vi "Unwrap Heading.vi"(11 "input":T1[](array[typedef])) -> (3 "output":T1[](array[typedef]))   [LabVIEW 2016]
uses:
  VIs/Segment.ctl
  <vilib>/ptbypt/NI_PtbyPt.lvlib
  Pathfinder.lvlib
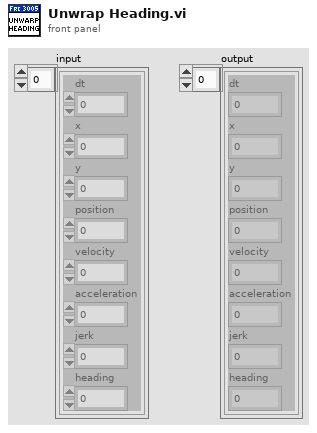
[diagram p1: front panel]
types:
  T1 = typedef "Pathfinder.lvlib/Segment.ctl" = cluster{"dt":dbl, "x":dbl, "y":dbl, "position":dbl, "velocity":dbl, "acceleration":dbl, "jerk":dbl, "heading":dbl}
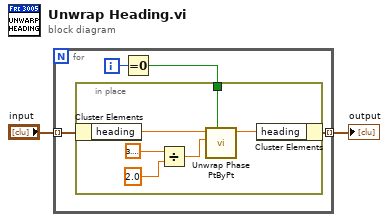
[diagram p0: block diagram]
diagram:
  n1 = for {
    tunnel: "input" -> [w6] mode=indexing
    tunnel: [w3] -> w2 mode=indexing
    i -> [w5]
    n2 = Equal To 0?(x=w5) -> (x = 0?=w4:bool)
    n3 = in-place {
      in-place-border: w4 -> [w9]
      n4 = in-place-cluster #1(w6) -> ("heading"=w12:dbl)
      n5 = Divide(x=3.141592653589793, y=2.0 ("x")) -> (x/y=w8:dbl)
      n6 = call <vilib>:"Unwrap Phase PtByPt.vi"("initialize"=w9, "wrap base"=w8, "phase"=w12) -> ("unwrapped phase"=w10:dbl)  [unwired: 8 in]
      n7 = in-place-cluster #1("heading"=w10) -> (w3:T1)
    }
  }
  "output" <- w2
